vi "Find Job Configuration File.vi"(8 "error in (no error)":errorcluster, 10 "Config.ext":string="xml", 11 "Job Folder":path) -> (0 "error out":errorcluster, 2 "Config File":path, 5 "Folder File Count":i32)   [LabVIEW 2015]
doc: "This vi is used to find the modeler configuration file within the job folder\n\nInputs\nJob Folder Path\nThe extension of the configuration file\n\nOutputs\nConfiguration Path (absolute)"
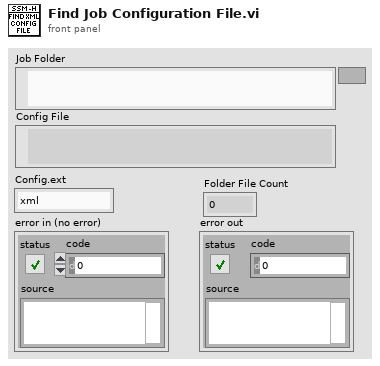
[diagram p1: front panel]
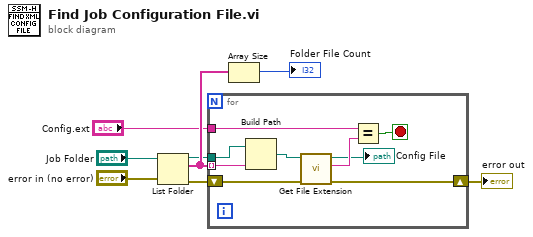
[diagram p0: block diagram]
diagram:
  n1 = List Folder(path="Job Folder", error in="error in (no error)") -> (path out=w4:path, filenames=w6:string[], error out=w3:errorcluster)  [unwired: 2 in, 1 out]
  n2 = for {
    tunnel: w6 -> [w17] mode=indexing
    tunnel: w4 -> [w16]
    shift-right: [w10] -> w7
    shift-left: w3 -> [w15]
    tunnel: "Config.ext" -> [w12]
    stop <- w11 stop-if-true
    n3 = Build Path(base path=w16, name or relative path=w17) -> (appended path=w14:path)
    n4 = call <vilib>:"Get File Extension.vi"("error in (no error)"=w15, "file"=w14) -> ("error out"=w10:errorcluster, "lowercase file extension"=w13:string, "dup file"=→"Config File":path)  [unwired: 5 in, 2 out]
    n5 = Equal?(x=w12, y=w13) -> (x = y?=w11:bool)
  }
  "error out" <- w7
  n6 = Array Size(array=w6) -> (size(s)=→"Folder File Count":i32)
